vi "solar_voy_def Import (cmd_tlm).vi"(6 "Suppress Errors? (T)":bool=TRUE, 8 "error in (no error)":errorcluster, 11 "cmd_tlm.txt":path) -> (0 "error out":errorcluster, 3 "PACKETS":T1[](array[typedef]) {"last_time" format="%<%H:%M:%S%3u %m/%d/%y>T"})   [LabVIEW 2018]
doc: "This imports a command or telemetry COSMOS file into packet definitions. Refer to http://cosmosrb.com/docs/cmdtlm/\n\nDefinition tags not supported: GENERIC_WRITE/READ_CONVERSION_START/END, MACRO_APPEND_START/END"
uses:
  solar_voy_def_ctl MODIFIERS STATE.ctl
  solar_voy_def_ctl MODIFIERS UNITS.ctl
  type/solar_type Item Type.ctl
  solar_voy_def_ctl ITEM TYPE.ctl
  solar_voy_def_ctl ITEM.ctl
  solar_voy_def_ctl PACKET_ID.ctl
  solar_voy_def_ctl PACKET.ctl
  solar_voy_def_ctl MODIFIERS LIMITS.ctl
  solar_voy_def_ctl MODIFIERS CONVERSION.ctl
  solar_voy_def_ctl MODIFIERS.ctl
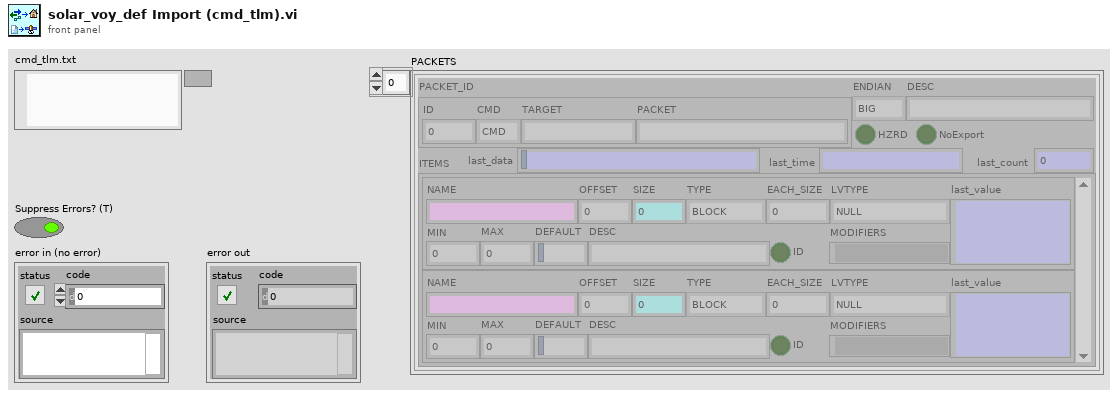
[diagram p1: front panel]
types:
  T1 = typedef "solar_voy_def_ctl PACKET.ctl" = cluster{"PACKET_ID":T2, "ENDIAN":enum8{"BIG", "LITTLE"}, "DESC":string, "HZRD":bool, "ITEMS":T3[], "NoExport":bool, "last_time":timestamp, "last_count":u32, "last_data":string}
  T2 = typedef "solar_voy_def_ctl PACKET_ID.ctl" = cluster{"ID":u16, "CMD":enum8{"CMD", "TLM"}, "TARGET":string, "PACKET":string}
  T3 = typedef "solar_voy_def_ctl ITEM.ctl" = cluster{"NAME":string, "OFFSET":i32, "SIZE":i32, "TYPE":T4, "EACH_SIZE":i32, "LVTYPE":T5, "MIN":dbl, "MAX":dbl, "DEFAULT":string, "DESC":string, "ID":bool, "MODIFIERS":variant, "last_value":variant}
  T4 = typedef "solar_voy_def_ctl ITEM TYPE.ctl" = enum8{"BLOCK", "INT", "UINT", "FLOAT", "STRING"}
  T5 = typedef "solar_type Item Type.ctl" = enum16{"NULL", "UNKNOWN", "CLUSTER", "I8", "I16", "I32", "I64", "U8", "U16", "U32", "U64", "U8_ENUM", "U16_ENUM", "U32_ENUM", "SGL", "DBL", "BOOLEAN", "STRING", "PATH", "VISA", "TAG", "TIME", "I8_1D", "I16_1D", "I32_1D", "I64_1D", "U8_1D", "U16_1D", "U32_1D", "U64_1D", "U8_ENUM_1D", "U16_ENUM_1D", "U32_ENUM_1D", "SGL_1D", "DBL_1D", "BOOLEAN_1D", "STRING_1D", "PATH_1D", "VISA_1D", "TAG_1D", "TIME_1D", "I8_2D", "I16_2D", "I32_2D", "I64_2D", "U8_2D", "U16_2D", "U32_2D", "U64_2D", "U8_ENUM_2D", "U16_ENUM_2D", "U32_ENUM_2D", "SGL_2D", "DBL_2D", "BOOLEAN_2D", "STRING_2D", "PATH_2D", "VISA_2D", "TAG_2D", "TIME_2D"}
  T6 = typedef "solar_voy_def_ctl MODIFIERS UNITS.ctl" = cluster{"FULL":string, "ABV":string}
  T7 = typedef "solar_voy_def_ctl MODIFIERS STATE.ctl" = cluster{"KEY":string, "VALUE":string, "COLOR":string, "DESC":string, "HZRD":bool}
  T8 = typedef "solar_voy_def_ctl MODIFIERS.ctl" = cluster{"LIMITS":T9, "UNITS":T6, "STATES":T7[], "CONVERSION":T10, "FORMAT":string, "REQUIRED":bool, "META":string[][]}
  T9 = typedef "solar_voy_def_ctl MODIFIERS LIMITS.ctl" = cluster{"NAME":string, "PERSIST":i32, "EN":bool, "RED_LO":dbl, "YEL_LO":dbl, "YEL_HI":dbl, "RED_HI":dbl, "GRN_LO":dbl, "GRN_HI":dbl, "FILENAME":string, "ARGS":string}
  T10 = typedef "solar_voy_def_ctl MODIFIERS CONVERSION.ctl" = cluster{"GENERIC":string, "FILENAME":string, "ARGS":string, "POLYS":cluster{"SEG":bool, "POLY":dbl[]}[]}
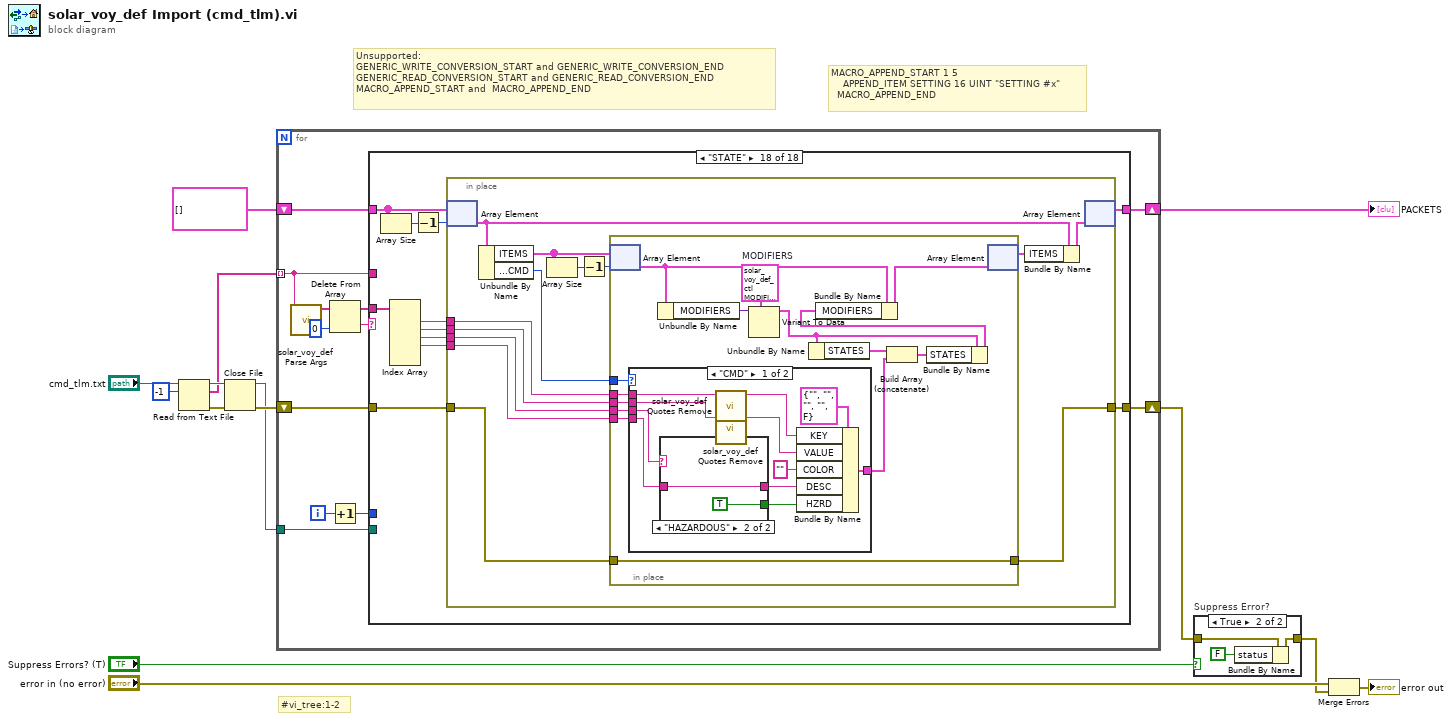
[diagram p0: block diagram]
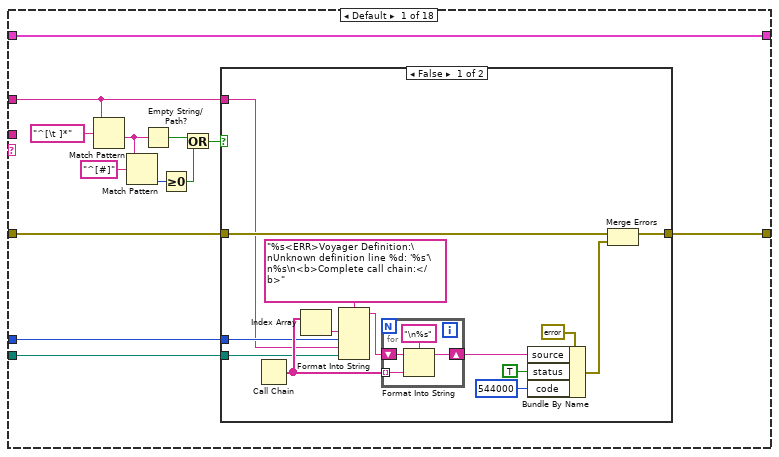
[diagram p2: hidden frame]
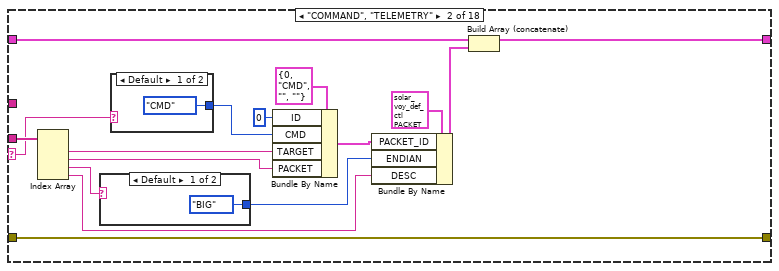
[diagram p4: hidden frame]
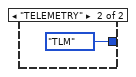
[diagram p5: hidden frame]
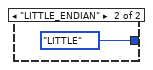
[diagram p6: hidden frame]
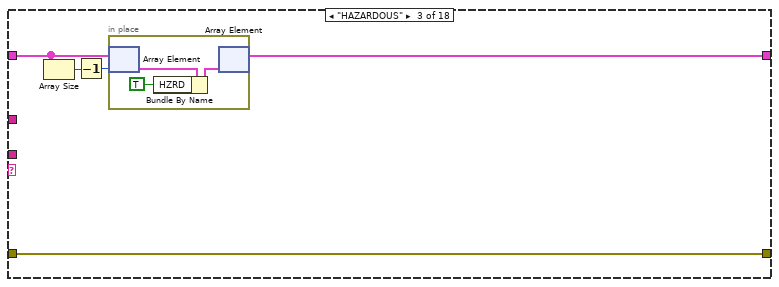
[diagram p7: hidden frame]
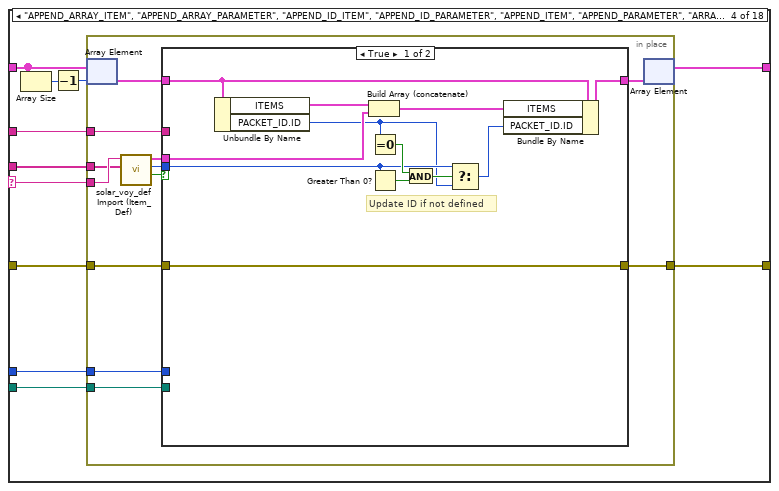
[diagram p8: hidden frame]
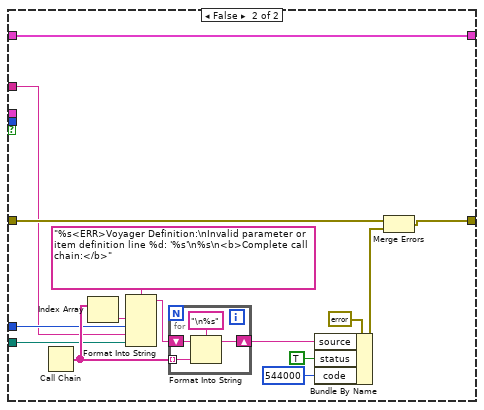
[diagram p9: hidden frame]
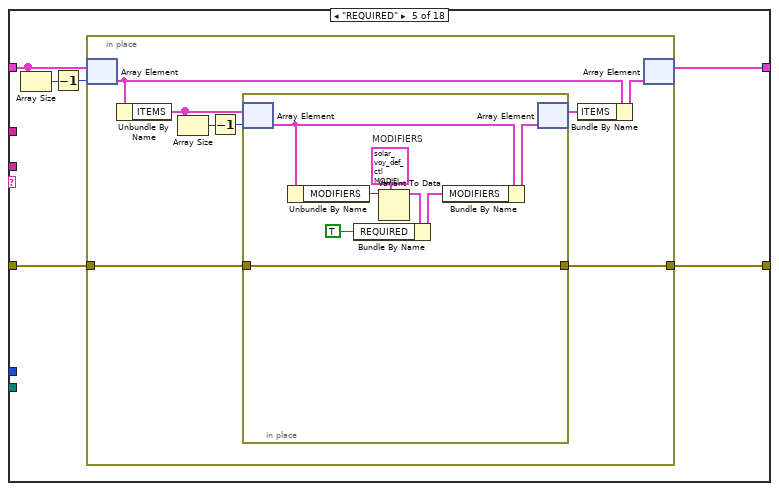
[diagram p10: hidden frame]
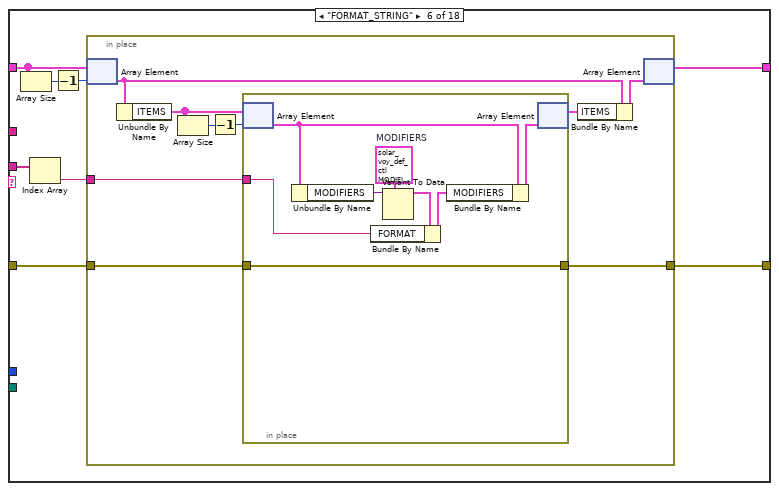
[diagram p11: hidden frame]
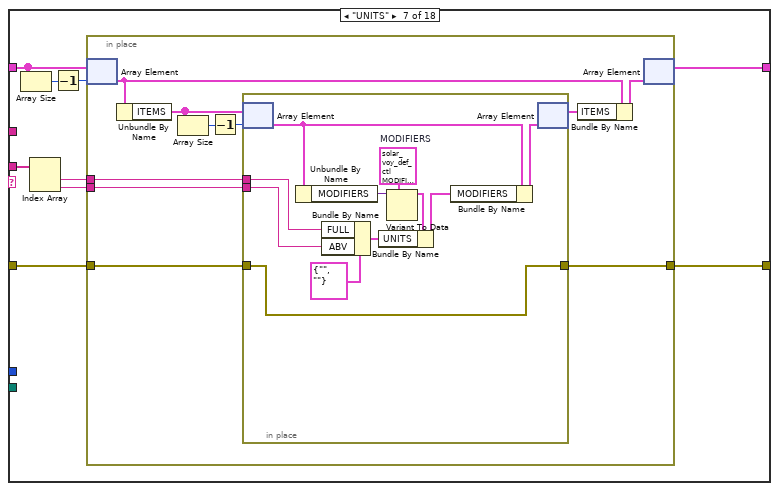
[diagram p12: hidden frame]
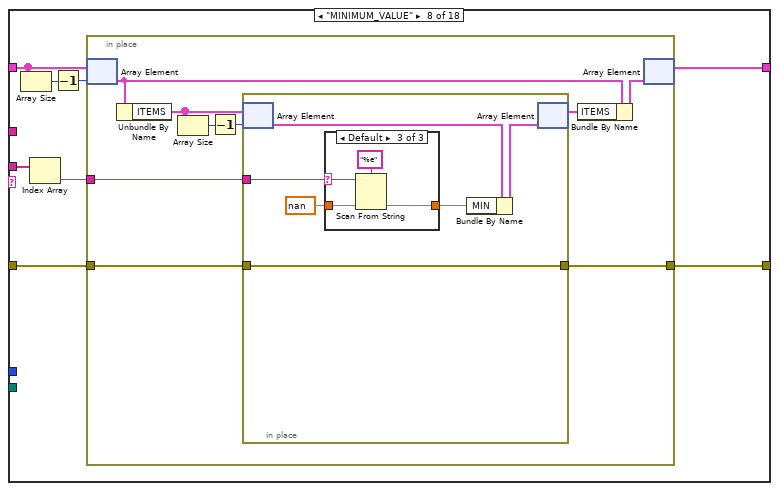
[diagram p13: hidden frame]
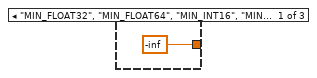
[diagram p14: hidden frame]
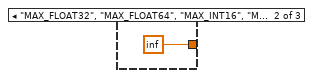
[diagram p15: hidden frame]
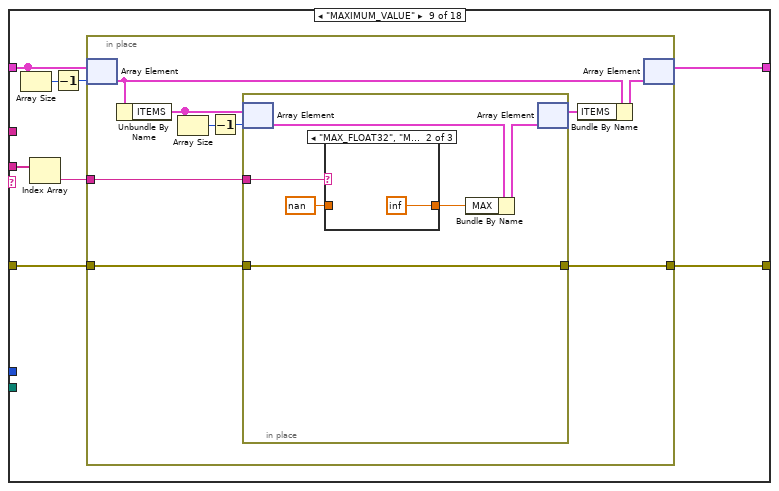
[diagram p16: hidden frame]
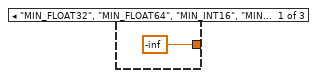
[diagram p17: hidden frame]
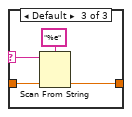
[diagram p18: hidden frame]
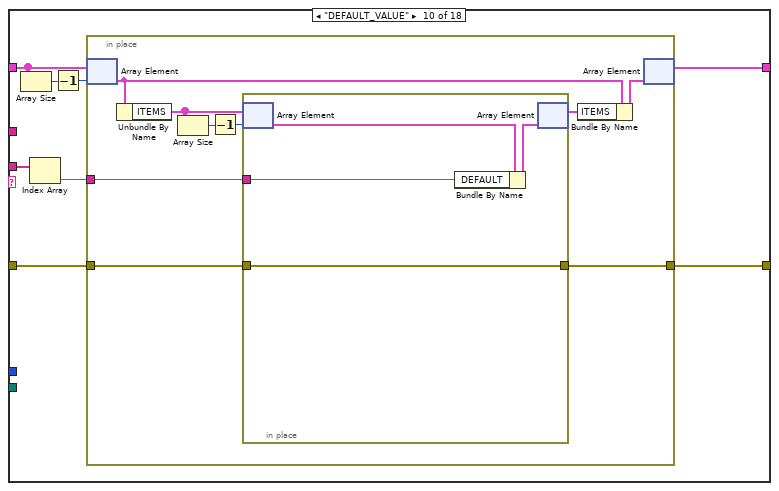
[diagram p19: hidden frame]
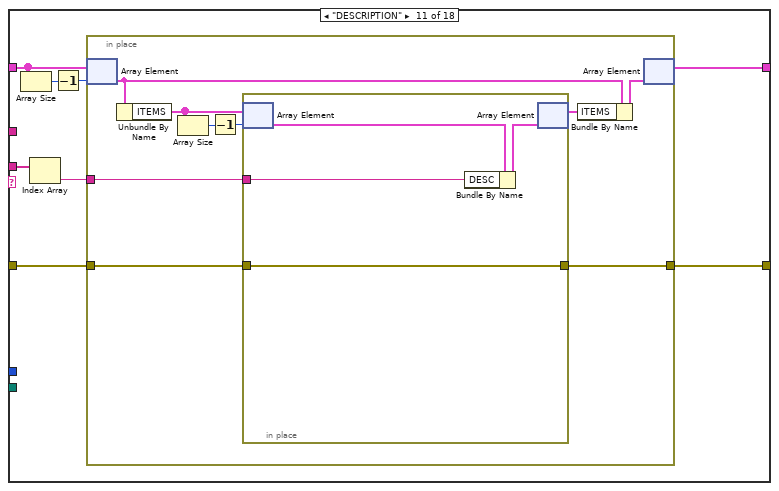
[diagram p20: hidden frame]
diagram:
  # "#vi_tree:1-2"
  # "MACRO_APPEND_START 1 5\n    APPEND_ITEM SETTING 16 UINT \"SETTING #x\"\n  MACRO_APPEND_END"
  # "Unsupported:\nGENERIC_WRITE_CONVERSION_START and GENERIC_WRITE_CONVERSION_END\nGENERIC_READ_CONVERSION_START and GENERIC_READ_CONVERSION_END\nMACRO_APPEND_START and  MACRO_APPEND_END"
  n1 = Read from Text File(file (use dialog)="cmd_tlm.txt", count=-1) -> (refnum out=w8:refnum<file>, text=w6:string[], error out=w7:errorcluster)  [unwired: 2 in, 1 out]
  n2 = Close File(refnum=w8, error in=w7) -> (path=w1:path, error out=w2:errorcluster)
  n3 = for {
    tunnel: w6 -> [w24] mode=indexing
    shift-right: [w26] -> w4
    shift-left: T1[] [] ("PACKETS") -> [w25]
    shift-right: [w23] -> w3
    shift-left: w2 -> [w22]
    tunnel: w1 -> [w17]
    i -> [w16]
    n4 = call "solar_voy_def Parse Args.vi"("String"=w24) -> ("Arguments"=w21:string[])  [unwired: 10 in]
    n5 = Delete From Array(array=w21, index=0) -> (deleted portion=w19:string, array with subset deleted=w18:string[])  [unwired: 1 in]
    n6 = Increment(x=w16) -> (x+1=w15:i32)
    n7 = case shown="\"STATE\"" w19 {
      selector: w19 -> [_ w59 _ w92 _ _ _ _ _ _ _ _ _ _ _ _ _ _]
      tunnel: [w39 w71 w80 w94 w143 w167 w193 w222 w251 w280 w301 w324 w355 w398 w452 w483 w517 w547] -> w26
      tunnel: w25 -> [w39 w72 w83 w97 w146 w170 w196 w225 w254 w283 w304 w327 w358 w401 w455 w486 w520 w550]
      tunnel: w24 -> [w34 _ _ w89 _ _ _ _ _ _ _ _ _ _ _ _ _ _]
      tunnel: [w36 w74 w79 w90 w141 w165 w191 w220 w249 w278 w299 w322 w353 w396 w450 w481 w515 w545] -> w23
      tunnel: w22 -> [w35 w74 w79 w91 w142 w166 w192 w221 w250 w279 w300 w323 w354 w397 w451 w482 w516 w546]
      tunnel: w18 -> [_ w73 _ w93 _ w164 w190 w219 w248 w277 w298 w321 w352 w395 w448 w480 w514 w544]
      tunnel: w17 -> [w38 _ _ w88 _ _ _ _ _ _ _ _ _ _ _ _ _ _]
      tunnel: w15 -> [w37 _ _ w87 _ _ _ _ _ _ _ _ _ _ _ _ _ _]
      frame Default {
        n8 = Match Pattern(string=w34, regular expression="^[\t ]*") -> (after substring=w31:string)  [unwired: 1 in, 3 out]
        n9 = Match Pattern(string=w31, regular expression="^[#]") -> (offset past match=w30:i32)  [unwired: 1 in, 3 out]
        n10 = Empty String/Path?(string/path=w31) -> (empty?=w29:bool)
        n11 = Greater Or Equal To 0?(x=w30) -> (x >= 0?=w28:bool)
        n12 = Or(x=w29, y=w28) -> (x .or. y?=w27:bool)
        n13 = case shown="False" w27 {
          tunnel: w38 -> [w44 _]
          tunnel: w37 -> [w43 _]
          tunnel: [w42 w58] -> w36
          tunnel: w35 -> [w41 w58]
          tunnel: w34 -> [w40 _]
          frame False {
            n14 = Call Chain() -> (call chain=w48:string[])
            n15 = Index Array(array=w48) -> (element=w50:string)  [unwired: 1 in]
            n16 = Format Into String(format string="%s<ERR>Voyager Definition:\nUnknown definition line %d: '%s'\n%s\n<b>Complete call chain:</b>", w50, w43, w40, w44) -> (resulting string=w49:string)  [unwired: 2 in, 1 out]
            n17 = for {
              tunnel: w48 -> [w57] mode=indexing
              shift-right: [w56] -> w47
              shift-left: w49 -> [w55]
              n18 = Format Into String(format string="\n%s", initial string=w55, w57) -> (resulting string=w56:string)  [unwired: 1 in, 1 out]
            }
            n19 = Bundle By Name(cluster=errorcluster {"status"=FALSE, "code"=0, "source"=""} ("error in (no error)"), "source"=w47, "status"=TRUE, "code"=544000 ("Code")) -> (w45:errorcluster)
            n20 = Merge Errors(w41, w45) -> (w42:errorcluster)
          }
          frame True {
            # "Empty line or comment\n- Ignore"
          }
        }
      }
      frame "COMMAND", "TELEMETRY" {
        n21 = Index Array(array=w73) -> (element #1=w70:string, element #2=w69:string, element #3=w68:string, element #4=w60:string)  [unwired: 4 in]
        n22 = case shown="Default" w68 {
          tunnel: [enum8{"BIG", "LITTLE"}."BIG" ("ENDIAN") enum8{"BIG", "LITTLE"}."LITTLE" ("ENDIAN")] -> w61
          frame Default {
          }
          frame "LITTLE_ENDIAN" {
          }
        }
        n23 = case shown="Default" w59 {
          tunnel: [enum8{"CMD", "TLM"}."CMD" ("PACKET_ID.CMD") enum8{"CMD", "TLM"}."TLM" ("PACKET_ID.CMD")] -> w67
          frame Default {
          }
          frame "TELEMETRY" {
          }
        }
        n24 = Bundle By Name(cluster=T2 {"ID"=0, "CMD"=enum."CMD", "TARGET"="", "PACKET"=""} ("PACKET_ID"), "ID"=u16 0, "CMD"=w67, "TARGET"=w70, "PACKET"=w69) -> (w62:T2)
        n25 = Bundle By Name(cluster=T1 {"PACKET_ID"={"ID"=0, "CMD"=enum."CMD", "TARGET"="", "PACKET"=""}, "ENDIAN"=enum."BIG", "DESC"="", "HZRD"=FALSE, "ITEMS"=[], "NoExport"=FALSE, "last_time"=timestamp(0 s since 1904-01-01), "last_count"=0, "last_data"=""} ("PACKET"), "PACKET_ID"=w62, "ENDIAN"=w61, "DESC"=w60) -> (w63:T1)
        n26 = Build Array (concatenate)(w72, w63) -> (w71:T1[])
      }
      frame "HAZARDOUS" {
        n27 = Array Size(array=w83) -> (size(s)=w82:i32)
        n28 = Decrement(x=w82) -> (x-1=w81:i32)
        n29 = in-place {
          n30 = in-place-array #1(w83, w81) -> (w86:T1)
          n31 = Bundle By Name(cluster=w86, "HZRD"=TRUE) -> (w85:T1)
          n32 = in-place-array #1(w85) -> (w80:T1[])  [unwired: 1 out]
        }
      }
      frame "APPEND_ARRAY_ITEM", "APPEND_ARRAY_PARAMETER", "APPEND_ID_ITEM", "APPEND_ID_PARAMETER", "APPEND_ITEM", "APPEND_PARAMETER", "ARRAY_ITEM", "ARRAY_PARAMETER", "ID_ITEM", "ID_PARAMETER", "ITEM", "PARAMETER" {
        n33 = Array Size(array=w97) -> (size(s)=w96:i32)
        n34 = Decrement(x=w96) -> (x-1=w95:i32)
        n35 = in-place {
          in-place-border: w93 -> [w105]
          in-place-border: w92 -> [w106]
          in-place-border: [w103] -> w90
          in-place-border: w91 -> [w102]
          in-place-border: w89 -> [w101]
          in-place-border: w88 -> [w100]
          in-place-border: w87 -> [w99]
          n36 = in-place-array #2(w97, w95) -> (w109:T1)
          n37 = call "solar_voy_def Import (Item_Def).vi"("Arguments"=w105, "Item Tag"=w106) -> ("Valid?"=w104:bool, "ID"=w98:u16, "ITEM"=w107:T3)  [unwired: 7 in]
          n38 = case shown="True" w104 {
            tunnel: w109 -> [w121 w125]
            tunnel: [w120 w125] -> w108
            tunnel: w107 -> [w117 _]
            tunnel: [w110 w127] -> w103
            tunnel: w102 -> [w110 w136]
            tunnel: w101 -> [_ w123]
            tunnel: w100 -> [_ w122]
            tunnel: w99 -> [_ w124]
            tunnel: w98 -> [w113 _]
            frame True {
              # "Update ID if not defined"
              n39 = Unbundle By Name(w121) -> ("ITEMS"=w119:T3[], "PACKET_ID.ID"=w112:u16)
              n40 = Build Array (concatenate)(w119, w117) -> (w118:T3[])
              n41 = Equal To 0?(x=w112) -> (x = 0?=w116:bool)
              n42 = Greater Than 0?(x=w113) -> (x > 0?=w115:bool)
              n43 = And(x=w116, y=w115) -> (x .and. y?=w114:bool)
              n44 = Select(t=w113, s=w114, f=w112) -> (s? t:f=w111:u16)
              n45 = Bundle By Name(cluster=w121, "ITEMS"=w118, "PACKET_ID.ID"=w111) -> (w120:T1)
            }
            frame False {
              n46 = Call Chain() -> (call chain=w130:string[])
              n47 = Index Array(array=w130) -> (element=w132:string)  [unwired: 1 in]
              n48 = Format Into String(format string="%s<ERR>Voyager Definition:\nInvalid parameter or item definition line %d: '%s'\n%s\n<b>Complete call chain:</b>", w132, w124, w123, w122) -> (resulting string=w131:string)  [unwired: 2 in, 1 out]
              n49 = for {
                tunnel: w130 -> [w140] mode=indexing
                shift-right: [w139] -> w129
                shift-left: w131 -> [w138]
                n50 = Format Into String(format string="\n%s", initial string=w138, w140) -> (resulting string=w139:string)  [unwired: 1 in, 1 out]
              }
              n51 = Bundle By Name(cluster=errorcluster {"status"=FALSE, "code"=0, "source"=""} ("error in (no error)"), "source"=w129, "status"=TRUE, "code"=544000 ("Code")) -> (w126:errorcluster)
              n52 = Merge Errors(w136, w126) -> (w127:errorcluster)
            }
          }
          n53 = in-place-array #2(w108) -> (w94:T1[])  [unwired: 1 out]
        }
      }
      frame "REQUIRED" {
        n54 = Array Size(array=w146) -> (size(s)=w145:i32)
        n55 = Decrement(x=w145) -> (x-1=w144:i32)
        n56 = in-place {
          in-place-border: [w148] -> w141
          in-place-border: w142 -> [w147]
          n57 = in-place-array #3(w146, w144) -> (w154:T1)
          n58 = Unbundle By Name(w154) -> ("ITEMS"=w151:T3[])
          n59 = Array Size(array=w151) -> (size(s)=w152:i32)
          n60 = Decrement(x=w152) -> (x-1=w150:i32)
          n61 = in-place {
            in-place-border: [w161] -> w148
            in-place-border: w147 -> [w161]
            w158 = T8 {"LIMITS"={"NAME"="", "PERSIST"=0, "EN"=FALSE, "RED_LO"=0.0, "YEL_LO"=0.0, "YEL_HI"=0.0, "RED_HI"=0.0, "GRN_LO"=0.0, "GRN_HI"=0.0, "FILENAME"="", "ARGS"=""}, "UNITS"={"FULL"="", "ABV"=""}, "STATES"=[], "CONVERSION"={"GENERIC"="", "FILENAME"="", "ARGS"="", "POLYS"=[]}, "FORMAT"="", "REQUIRED"=FALSE, "META"=[]}  # MODIFIERS
            n62 = in-place-array #4(w151, w150) -> (w156:T3)
            n63 = Unbundle By Name(w156) -> ("MODIFIERS"=w159:variant)
            n64 = Variant To Data(type=w158, Variant=w159) -> (data=w157:T8)  [unwired: 1 in, 1 out]
            n65 = Bundle By Name(cluster=w157, "REQUIRED"=TRUE ("MODIFIERS.REQUIRED")) -> (w155:T8)
            n66 = Bundle By Name(cluster=w156, "MODIFIERS"=w155) -> (w160:T3)
            n67 = in-place-array #4(w160) -> (w149:T3[])  [unwired: 1 out]
          }
          n68 = Bundle By Name(cluster=w154, "ITEMS"=w149) -> (w153:T1)
          n69 = in-place-array #3(w153) -> (w143:T1[])  [unwired: 1 out]
        }
      }
      frame "FORMAT_STRING" {
        n70 = Array Size(array=w170) -> (size(s)=w169:i32)
        n71 = Index Array(array=w164) -> (element=w163:string)  [unwired: 1 in]
        n72 = Decrement(x=w169) -> (x-1=w168:i32)
        n73 = in-place {
          in-place-border: [w173] -> w165
          in-place-border: w166 -> [w172]
          in-place-border: w163 -> [w171]
          n74 = in-place-array #5(w170, w168) -> (w179:T1)
          n75 = Unbundle By Name(w179) -> ("ITEMS"=w176:T3[])
          n76 = Array Size(array=w176) -> (size(s)=w177:i32)
          n77 = Decrement(x=w177) -> (x-1=w175:i32)
          n78 = in-place {
            in-place-border: [w187] -> w173
            in-place-border: w172 -> [w187]
            in-place-border: w171 -> [w186]
            w184 = T8 {"LIMITS"={"NAME"="", "PERSIST"=0, "EN"=FALSE, "RED_LO"=0.0, "YEL_LO"=0.0, "YEL_HI"=0.0, "RED_HI"=0.0, "GRN_LO"=0.0, "GRN_HI"=0.0, "FILENAME"="", "ARGS"=""}, "UNITS"={"FULL"="", "ABV"=""}, "STATES"=[], "CONVERSION"={"GENERIC"="", "FILENAME"="", "ARGS"="", "POLYS"=[]}, "FORMAT"="", "REQUIRED"=FALSE, "META"=[]}  # MODIFIERS
            n79 = in-place-array #6(w176, w175) -> (w182:T3)
            n80 = Unbundle By Name(w182) -> ("MODIFIERS"=w185:variant)
            n81 = Variant To Data(type=w184, Variant=w185) -> (data=w181:T8)  [unwired: 1 in, 1 out]
            n82 = Bundle By Name(cluster=w181, "FORMAT"=w186) -> (w180:T8)
            n83 = Bundle By Name(cluster=w182, "MODIFIERS"=w180) -> (w183:T3)
            n84 = in-place-array #6(w183) -> (w174:T3[])  [unwired: 1 out]
          }
          n85 = Bundle By Name(cluster=w179, "ITEMS"=w174) -> (w178:T1)
          n86 = in-place-array #5(w178) -> (w167:T1[])  [unwired: 1 out]
        }
      }
      frame "UNITS" {
        n87 = Array Size(array=w196) -> (size(s)=w195:i32)
        n88 = Index Array(array=w190) -> (element #1=w189:string, element #2=w188:string)  [unwired: 2 in]
        n89 = Decrement(x=w195) -> (x-1=w194:i32)
        n90 = in-place {
          in-place-border: [w200] -> w191
          in-place-border: w192 -> [w199]
          in-place-border: w189 -> [w198]
          in-place-border: w188 -> [w197]
          n91 = in-place-array #7(w196, w194) -> (w206:T1)
          n92 = Unbundle By Name(w206) -> ("ITEMS"=w203:T3[])
          n93 = Array Size(array=w203) -> (size(s)=w204:i32)
          n94 = Decrement(x=w204) -> (x-1=w202:i32)
          n95 = in-place {
            in-place-border: [w207] -> w200
            in-place-border: w199 -> [w207]
            in-place-border: w198 -> [w216]
            in-place-border: w197 -> [w215]
            w212 = T8 {"LIMITS"={"NAME"="", "PERSIST"=0, "EN"=FALSE, "RED_LO"=0.0, "YEL_LO"=0.0, "YEL_HI"=0.0, "RED_HI"=0.0, "GRN_LO"=0.0, "GRN_HI"=0.0, "FILENAME"="", "ARGS"=""}, "UNITS"={"FULL"="", "ABV"=""}, "STATES"=[], "CONVERSION"={"GENERIC"="", "FILENAME"="", "ARGS"="", "POLYS"=[]}, "FORMAT"="", "REQUIRED"=FALSE, "META"=[]}  # MODIFIERS
            n96 = in-place-array #8(w203, w202) -> (w211:T3)
            n97 = Unbundle By Name(w211) -> ("MODIFIERS"=w213:variant)
            n98 = Bundle By Name(cluster=T6 {"FULL"="", "ABV"=""} ("MODIFIERS.UNITS"), "FULL"=w216, "ABV"=w215) -> (w214:T6)
            n99 = Variant To Data(type=w212, Variant=w213) -> (data=w209:T8)  [unwired: 1 in, 1 out]
            n100 = Bundle By Name(cluster=w209, "UNITS"=w214) -> (w208:T8)
            n101 = Bundle By Name(cluster=w211, "MODIFIERS"=w208) -> (w210:T3)
            n102 = in-place-array #8(w210) -> (w201:T3[])  [unwired: 1 out]
          }
          n103 = Bundle By Name(cluster=w206, "ITEMS"=w201) -> (w205:T1)
          n104 = in-place-array #7(w205) -> (w193:T1[])  [unwired: 1 out]
        }
      }
      frame "MINIMUM_VALUE" {
        n105 = Array Size(array=w225) -> (size(s)=w224:i32)
        n106 = Index Array(array=w219) -> (element=w218:string)  [unwired: 1 in]
        n107 = Decrement(x=w224) -> (x-1=w223:i32)
        n108 = in-place {
          in-place-border: [w228] -> w220
          in-place-border: w221 -> [w227]
          in-place-border: w218 -> [w226]
          n109 = in-place-array #9(w225, w223) -> (w234:T1)
          n110 = Unbundle By Name(w234) -> ("ITEMS"=w231:T3[])
          n111 = Array Size(array=w231) -> (size(s)=w232:i32)
          n112 = Decrement(x=w232) -> (x-1=w230:i32)
          n113 = in-place {
            in-place-border: [w238] -> w228
            in-place-border: w227 -> [w238]
            in-place-border: w226 -> [w237]
            n114 = in-place-array #10(w231, w230) -> (w240:T3)
            n115 = case shown="Default" w237 {
              selector: w237 -> [_ _ w246]
              tunnel: nan ("MIN") -> [_ _ w245]
              tunnel: [-inf ("MIN") inf ("MIN") w244] -> w235
              frame "MIN_FLOAT32", "MIN_FLOAT64", "MIN_INT16", "MIN_INT32", "MIN_INT64", "MIN_INT8", "MIN_UINT16", "MIN_UINT32", "MIN_UINT64", "MIN_UINT8" {
              }
              frame "MAX_FLOAT32", "MAX_FLOAT64", "MAX_INT16", "MAX_INT32", "MAX_INT64", "MAX_INT8", "MAX_UINT16", "MAX_UINT32", "MAX_UINT64", "MAX_UINT8" {
              }
              frame Default {
                n116 = Scan From String(format string="%e", input string=w246, default 1=w245) -> (output 1=w244:dbl)  [unwired: 2 in, 3 out]
              }
            }
            n117 = Bundle By Name(cluster=w240, "MIN"=w235) -> (w239:T3)
            n118 = in-place-array #10(w239) -> (w229:T3[])  [unwired: 1 out]
          }
          n119 = Bundle By Name(cluster=w234, "ITEMS"=w229) -> (w233:T1)
          n120 = in-place-array #9(w233) -> (w222:T1[])  [unwired: 1 out]
        }
      }
      frame "MAXIMUM_VALUE" {
        n121 = Array Size(array=w254) -> (size(s)=w253:i32)
        n122 = Index Array(array=w248) -> (element=w247:string)  [unwired: 1 in]
        n123 = Decrement(x=w253) -> (x-1=w252:i32)
        n124 = in-place {
          in-place-border: [w257] -> w249
          in-place-border: w250 -> [w256]
          in-place-border: w247 -> [w255]
          n125 = in-place-array #11(w254, w252) -> (w263:T1)
          n126 = Unbundle By Name(w263) -> ("ITEMS"=w260:T3[])
          n127 = Array Size(array=w260) -> (size(s)=w261:i32)
          n128 = Decrement(x=w261) -> (x-1=w259:i32)
          n129 = in-place {
            in-place-border: [w267] -> w257
            in-place-border: w256 -> [w267]
            in-place-border: w255 -> [w266]
            n130 = in-place-array #12(w260, w259) -> (w269:T3)
            n131 = case shown="\"MAX_FLOAT32\", \"MAX_FLOAT64\", \"MAX_INT16\", \"MAX_INT32\", \"MAX_INT64\", \"MAX_INT8\", \"MAX_UINT16\", \"MAX_UINT32\", \"MAX_UINT64\", \"MAX_UINT8\"" w266 {
              selector: w266 -> [_ _ w275]
              tunnel: nan ("MIN") -> [_ _ w274]
              tunnel: [-inf ("MIN") inf ("MIN") w273] -> w264
              frame "MIN_FLOAT32", "MIN_FLOAT64", "MIN_INT16", "MIN_INT32", "MIN_INT64", "MIN_INT8", "MIN_UINT16", "MIN_UINT32", "MIN_UINT64", "MIN_UINT8" {
              }
              frame "MAX_FLOAT32", "MAX_FLOAT64", "MAX_INT16", "MAX_INT32", "MAX_INT64", "MAX_INT8", "MAX_UINT16", "MAX_UINT32", "MAX_UINT64", "MAX_UINT8" {
              }
              frame Default {
                n132 = Scan From String(format string="%e", input string=w275, default 1=w274) -> (output 1=w273:dbl)  [unwired: 2 in, 3 out]
              }
            }
            n133 = Bundle By Name(cluster=w269, "MAX"=w264) -> (w268:T3)
            n134 = in-place-array #12(w268) -> (w258:T3[])  [unwired: 1 out]
          }
          n135 = Bundle By Name(cluster=w263, "ITEMS"=w258) -> (w262:T1)
          n136 = in-place-array #11(w262) -> (w251:T1[])  [unwired: 1 out]
        }
      }
      frame "DEFAULT_VALUE" {
        n137 = Array Size(array=w283) -> (size(s)=w282:i32)
        n138 = Index Array(array=w277) -> (element=w276:string)  [unwired: 1 in]
        n139 = Decrement(x=w282) -> (x-1=w281:i32)
        n140 = in-place {
          in-place-border: [w286] -> w278
          in-place-border: w279 -> [w285]
          in-place-border: w276 -> [w284]
          n141 = in-place-array #13(w283, w281) -> (w292:T1)
          n142 = Unbundle By Name(w292) -> ("ITEMS"=w289:T3[])
          n143 = Array Size(array=w289) -> (size(s)=w290:i32)
          n144 = Decrement(x=w290) -> (x-1=w288:i32)
          n145 = in-place {
            in-place-border: [w294] -> w286
            in-place-border: w285 -> [w294]
            in-place-border: w284 -> [w293]
            n146 = in-place-array #14(w289, w288) -> (w296:T3)
            n147 = Bundle By Name(cluster=w296, "DEFAULT"=w293) -> (w295:T3)
            n148 = in-place-array #14(w295) -> (w287:T3[])  [unwired: 1 out]
          }
          n149 = Bundle By Name(cluster=w292, "ITEMS"=w287) -> (w291:T1)
          n150 = in-place-array #13(w291) -> (w280:T1[])  [unwired: 1 out]
        }
      }
      frame "DESCRIPTION" {
        n151 = Array Size(array=w304) -> (size(s)=w303:i32)
        n152 = Index Array(array=w298) -> (element=w297:string)  [unwired: 1 in]
        n153 = Decrement(x=w303) -> (x-1=w302:i32)
        n154 = in-place {
          in-place-border: [w307] -> w299
          in-place-border: w300 -> [w306]
          in-place-border: w297 -> [w305]
          n155 = in-place-array #15(w304, w302) -> (w313:T1)
          n156 = Unbundle By Name(w313) -> ("ITEMS"=w310:T3[])
          n157 = Array Size(array=w310) -> (size(s)=w311:i32)
          n158 = Decrement(x=w311) -> (x-1=w309:i32)
          n159 = in-place {
            in-place-border: [w315] -> w307
            in-place-border: w306 -> [w315]
            in-place-border: w305 -> [w314]
            n160 = in-place-array #16(w310, w309) -> (w317:T3)
            n161 = Bundle By Name(cluster=w317, "DESC"=w314) -> (w316:T3)
            n162 = in-place-array #16(w316) -> (w308:T3[])  [unwired: 1 out]
          }
          n163 = Bundle By Name(cluster=w313, "ITEMS"=w308) -> (w312:T1)
          n164 = in-place-array #15(w312) -> (w301:T1[])  [unwired: 1 out]
        }
      }
      frame "READ_CONVERSION", "WRITE_CONVERSION" {
        n165 = Array Size(array=w327) -> (size(s)=w326:i32)
        n166 = Delete From Array(array=w321, index=0) -> (deleted portion=w320:string, array with subset deleted=w318:string[])  [unwired: 1 in]
        n167 = Decrement(x=w326) -> (x-1=w325:i32)
        n168 = in-place {
          in-place-border: [w333] -> w322
          in-place-border: w323 -> [w332]
          in-place-border: w320 -> [w331]
          in-place-border: w318 -> [w330]
          n169 = in-place-array #17(w327, w325) -> (w339:T1)
          n170 = for {
            tunnel: w330 -> [w342] mode=indexing
            tunnel: [w340] -> w329 mode=indexing
            n171 = Concatenate Strings(w342, " " ("string")) -> (w340:string)
          }
          n172 = Unbundle By Name(w339) -> ("ITEMS"=w336:T3[])
          n173 = Array Size(array=w336) -> (size(s)=w337:i32)
          n174 = Decrement(x=w337) -> (x-1=w335:i32)
          n175 = Concatenate Strings(w329) -> (w328:string)
          n176 = in-place {
            in-place-border: [w351] -> w333
            in-place-border: w332 -> [w351]
            in-place-border: w331 -> [w350]
            in-place-border: w328 -> [w349]
            w347 = T8 {"LIMITS"={"NAME"="", "PERSIST"=0, "EN"=FALSE, "RED_LO"=0.0, "YEL_LO"=0.0, "YEL_HI"=0.0, "RED_HI"=0.0, "GRN_LO"=0.0, "GRN_HI"=0.0, "FILENAME"="", "ARGS"=""}, "UNITS"={"FULL"="", "ABV"=""}, "STATES"=[], "CONVERSION"={"GENERIC"="", "FILENAME"="", "ARGS"="", "POLYS"=[]}, "FORMAT"="", "REQUIRED"=FALSE, "META"=[]}  # MODIFIERS
            n177 = in-place-array #18(w336, w335) -> (w346:T3)
            n178 = Unbundle By Name(w346) -> ("MODIFIERS"=w348:variant)
            n179 = Variant To Data(type=w347, Variant=w348) -> (data=w344:T8)  [unwired: 1 in, 1 out]
            n180 = Bundle By Name(cluster=w344, "CONVERSION.FILENAME"=w350, "CONVERSION.ARGS"=w349) -> (w343:T8)
            n181 = Bundle By Name(cluster=w346, "MODIFIERS"=w343) -> (w345:T3)
            n182 = in-place-array #18(w345) -> (w334:T3[])  [unwired: 1 out]
          }
          n183 = Bundle By Name(cluster=w339, "ITEMS"=w334) -> (w338:T1)
          n184 = in-place-array #17(w338) -> (w324:T1[])  [unwired: 1 out]
        }
      }
      frame "SEG_POLY_READ_CONVERSION", "SEG_POLY_WRITE_CONVERSION" {
        n185 = Array Size(array=w358) -> (size(s)=w357:i32)
        n186 = Decrement(x=w357) -> (x-1=w356:i32)
        n187 = in-place {
          in-place-border: [w362] -> w353
          in-place-border: w354 -> [w361]
          in-place-border: w352 -> [w360]
          n188 = in-place-array #19(w358, w356) -> (w368:T1)
          n189 = for {
            tunnel: w360 -> [w372] mode=indexing
            tunnel: [w369] -> w359 mode=indexing
            n190 = Scan From String(format string="%e", input string=w372, default 1=nan ("default value 1")) -> (output 1=w369:dbl)  [unwired: 2 in, 3 out]
          }
          n191 = Unbundle By Name(w368) -> ("ITEMS"=w365:T3[])
          n192 = Array Size(array=w365) -> (size(s)=w366:i32)
          n193 = Decrement(x=w366) -> (x-1=w364:i32)
          n194 = in-place {
            in-place-border: [w379] -> w362
            in-place-border: w361 -> [w379]
            in-place-border: w359 -> [w380]
            w377 = T8 {"LIMITS"={"NAME"="", "PERSIST"=0, "EN"=FALSE, "RED_LO"=0.0, "YEL_LO"=0.0, "YEL_HI"=0.0, "RED_HI"=0.0, "GRN_LO"=0.0, "GRN_HI"=0.0, "FILENAME"="", "ARGS"=""}, "UNITS"={"FULL"="", "ABV"=""}, "STATES"=[], "CONVERSION"={"GENERIC"="", "FILENAME"="", "ARGS"="", "POLYS"=[]}, "FORMAT"="", "REQUIRED"=FALSE, "META"=[]}  # MODIFIERS
            n195 = in-place-array #20(w365, w364) -> (w376:T3)
            n196 = Unbundle By Name(w376) -> ("MODIFIERS"=w378:variant)
            n197 = Bundle By Name(cluster=cluster{"SEG":bool, "POLY":dbl[]} {"SEG"=FALSE, "POLY"=[]} ("POLY"), "SEG"=TRUE, "POLY"=w380) -> (w382:cluster{"SEG":bool, "POLY":dbl[]})
            n198 = Variant To Data(type=w377, Variant=w378) -> (data=w374:T8)  [unwired: 1 in, 1 out]
            n199 = Unbundle By Name(w374) -> ("CONVERSION.POLYS"=w385:cluster{"SEG":bool, "POLY":dbl[]}[])
            n200 = Build Array (concatenate)(w385, w382) -> (w384:cluster{"SEG":bool, "POLY":dbl[]}[])
            n201 = Bundle By Name(cluster=w374, "CONVERSION.POLYS"=w384) -> (w373:T8)
            n202 = Bundle By Name(cluster=w376, "MODIFIERS"=w373) -> (w375:T3)
            n203 = in-place-array #20(w375) -> (w363:T3[])  [unwired: 1 out]
          }
          n204 = Bundle By Name(cluster=w368, "ITEMS"=w363) -> (w367:T1)
          n205 = in-place-array #19(w367) -> (w355:T1[])  [unwired: 1 out]
        }
      }
      frame "LIMITS" {
        n206 = Array Size(array=w401) -> (size(s)=w400:i32)
        n207 = Index Array(array=w395) -> (element #1=w394:string, element #2=w393:string, element #3=w392:string, element #4=w391:string, element #5=w390:string, element #6=w389:string, element #7=w388:string, element #8=w387:string, element #9=w386:string)  [unwired: 9 in]
        n208 = Decrement(x=w400) -> (x-1=w399:i32)
        n209 = in-place {
          in-place-border: [w414] -> w396
          in-place-border: w397 -> [w413]
          in-place-border: w394 -> [w412]
          in-place-border: w393 -> [w411]
          in-place-border: w392 -> [w410]
          in-place-border: w391 -> [w409]
          in-place-border: w390 -> [w408]
          in-place-border: w389 -> [w407]
          in-place-border: w388 -> [w406]
          in-place-border: w387 -> [w405]
          in-place-border: w386 -> [w404]
          n210 = in-place-array #21(w401, w399) -> (w420:T1)
          n211 = Build Array(w409, w408, w407, w406, w405, w404) -> (w403:string[])
          n212 = Unbundle By Name(w420) -> ("ITEMS"=w417:T3[])
          n213 = for {
            tunnel: w403 -> [w424] mode=indexing
            tunnel: [w421] -> w402 mode=indexing
            n214 = Scan From String(format string="%e", input string=w424, default 1=nan ("default value 1")) -> (output 1=w421:dbl)  [unwired: 2 in, 3 out]
          }
          n215 = Array Size(array=w417) -> (size(s)=w418:i32)
          n216 = Decrement(x=w418) -> (x-1=w416:i32)
          n217 = in-place {
            in-place-border: [w444] -> w414
            in-place-border: w413 -> [w444]
            in-place-border: w412 -> [w443]
            in-place-border: w411 -> [w442]
            in-place-border: w410 -> [w439]
            in-place-border: w402 -> [w437]
            w429 = T8 {"LIMITS"={"NAME"="", "PERSIST"=0, "EN"=FALSE, "RED_LO"=0.0, "YEL_LO"=0.0, "YEL_HI"=0.0, "RED_HI"=0.0, "GRN_LO"=0.0, "GRN_HI"=0.0, "FILENAME"="", "ARGS"=""}, "UNITS"={"FULL"="", "ABV"=""}, "STATES"=[], "CONVERSION"={"GENERIC"="", "FILENAME"="", "ARGS"="", "POLYS"=[]}, "FORMAT"="", "REQUIRED"=FALSE, "META"=[]}  # MODIFIERS
            n218 = in-place-array #22(w417, w416) -> (w428:T3)
            n219 = case shown="\"ENABLED\"" w439 {
              tunnel: [_ TRUE] -> w438
              frame Default {
              }
              frame "ENABLED" {
              }
            }
            n220 = Index Array(array=w437) -> (element #1=w436:dbl, element #2=w435:dbl, element #3=w434:dbl, element #4=w433:dbl, element #5=w432:dbl, element #6=w431:dbl)  [unwired: 6 in]
            n221 = Decimal String To Number(string=w442, default (0L)=0 ("MODIFIERS.LIMITS.PERSIST")) -> (number=w440:i32)  [unwired: 1 in, 1 out]
            n222 = Unbundle By Name(w428) -> ("MODIFIERS"=w430:variant)
            n223 = Variant To Data(type=w429, Variant=w430) -> (data=w426:T8)  [unwired: 1 in, 1 out]
            n224 = Bundle By Name(cluster=w426, "LIMITS.NAME"=w443, "LIMITS.PERSIST"=w440, "LIMITS.EN"=w438, "LIMITS.RED_LO"=w436, "LIMITS.YEL_LO"=w435, "LIMITS.YEL_HI"=w434, "LIMITS.RED_HI"=w433, "LIMITS.GRN_LO"=w432, "LIMITS.GRN_HI"=w431) -> (w425:T8)
            n225 = Bundle By Name(cluster=w428, "MODIFIERS"=w425) -> (w427:T3)
            n226 = in-place-array #22(w427) -> (w415:T3[])  [unwired: 1 out]
          }
          n227 = Bundle By Name(cluster=w420, "ITEMS"=w415) -> (w419:T1)
          n228 = in-place-array #21(w419) -> (w398:T1[])  [unwired: 1 out]
        }
      }
      frame "LIMITS_RESPONSE" {
        n229 = Array Size(array=w455) -> (size(s)=w454:i32)
        n230 = Delete From Array(array=w448, index=0) -> (deleted portion=w447:string, array with subset deleted=w446:string[])  [unwired: 1 in]
        n231 = Decrement(x=w454) -> (x-1=w453:i32)
        n232 = in-place {
          in-place-border: [w461] -> w450
          in-place-border: w451 -> [w460]
          in-place-border: w447 -> [w459]
          in-place-border: w446 -> [w457]
          n233 = in-place-array #23(w455, w453) -> (w467:T1)
          n234 = for {
            tunnel: w457 -> [w470] mode=indexing
            tunnel: [w468] -> w458 mode=indexing
            n235 = Concatenate Strings(w470, " " ("string")) -> (w468:string)
          }
          n236 = Unbundle By Name(w467) -> ("ITEMS"=w464:T3[])
          n237 = Array Size(array=w464) -> (size(s)=w465:i32)
          n238 = Decrement(x=w465) -> (x-1=w463:i32)
          n239 = Concatenate Strings(w458) -> (w456:string)
          n240 = in-place {
            in-place-border: [w479] -> w461
            in-place-border: w460 -> [w479]
            in-place-border: w459 -> [w478]
            in-place-border: w456 -> [w477]
            w475 = T8 {"LIMITS"={"NAME"="", "PERSIST"=0, "EN"=FALSE, "RED_LO"=0.0, "YEL_LO"=0.0, "YEL_HI"=0.0, "RED_HI"=0.0, "GRN_LO"=0.0, "GRN_HI"=0.0, "FILENAME"="", "ARGS"=""}, "UNITS"={"FULL"="", "ABV"=""}, "STATES"=[], "CONVERSION"={"GENERIC"="", "FILENAME"="", "ARGS"="", "POLYS"=[]}, "FORMAT"="", "REQUIRED"=FALSE, "META"=[]}  # MODIFIERS
            n241 = in-place-array #24(w464, w463) -> (w472:T3)
            n242 = Unbundle By Name(w472) -> ("MODIFIERS"=w476:variant)
            n243 = Variant To Data(type=w475, Variant=w476) -> (data=w474:T8)  [unwired: 1 in, 1 out]
            n244 = Bundle By Name(cluster=w474, "LIMITS.FILENAME"=w478, "LIMITS.ARGS"=w477) -> (w473:T8)
            n245 = Bundle By Name(cluster=w472, "MODIFIERS"=w473) -> (w471:T3)
            n246 = in-place-array #24(w471) -> (w462:T3[])  [unwired: 1 out]
          }
          n247 = Bundle By Name(cluster=w467, "ITEMS"=w462) -> (w466:T1)
          n248 = in-place-array #23(w466) -> (w452:T1[])  [unwired: 1 out]
        }
      }
      frame "POLY_READ_CONVERSION", "POLY_WRITE_CONVERSION" {
        n249 = Array Size(array=w486) -> (size(s)=w485:i32)
        n250 = Decrement(x=w485) -> (x-1=w484:i32)
        n251 = in-place {
          in-place-border: [w490] -> w481
          in-place-border: w482 -> [w489]
          in-place-border: w480 -> [w488]
          n252 = in-place-array #25(w486, w484) -> (w496:T1)
          n253 = for {
            tunnel: w488 -> [w500] mode=indexing
            tunnel: [w497] -> w487 mode=indexing
            n254 = Scan From String(format string="%e", input string=w500, default 1=nan ("default value 1")) -> (output 1=w497:dbl)  [unwired: 2 in, 3 out]
          }
          n255 = Unbundle By Name(w496) -> ("ITEMS"=w493:T3[])
          n256 = Array Size(array=w493) -> (size(s)=w494:i32)
          n257 = Decrement(x=w494) -> (x-1=w492:i32)
          n258 = in-place {
            in-place-border: [w507] -> w490
            in-place-border: w489 -> [w507]
            in-place-border: w487 -> [w508]
            w505 = T8 {"LIMITS"={"NAME"="", "PERSIST"=0, "EN"=FALSE, "RED_LO"=0.0, "YEL_LO"=0.0, "YEL_HI"=0.0, "RED_HI"=0.0, "GRN_LO"=0.0, "GRN_HI"=0.0, "FILENAME"="", "ARGS"=""}, "UNITS"={"FULL"="", "ABV"=""}, "STATES"=[], "CONVERSION"={"GENERIC"="", "FILENAME"="", "ARGS"="", "POLYS"=[]}, "FORMAT"="", "REQUIRED"=FALSE, "META"=[]}  # MODIFIERS
            n259 = in-place-array #26(w493, w492) -> (w504:T3)
            n260 = Unbundle By Name(w504) -> ("MODIFIERS"=w506:variant)
            n261 = Bundle By Name(cluster=cluster{"SEG":bool, "POLY":dbl[]} {"SEG"=FALSE, "POLY"=[]} ("POLY"), "SEG"=FALSE, "POLY"=w508) -> (w510:cluster{"SEG":bool, "POLY":dbl[]})
            n262 = Variant To Data(type=w505, Variant=w506) -> (data=w502:T8)  [unwired: 1 in, 1 out]
            n263 = Unbundle By Name(w502) -> ("CONVERSION.POLYS"=w513:cluster{"SEG":bool, "POLY":dbl[]}[])
            n264 = Build Array (concatenate)(w513, w510) -> (w512:cluster{"SEG":bool, "POLY":dbl[]}[])
            n265 = Bundle By Name(cluster=w502, "CONVERSION.POLYS"=w512) -> (w501:T8)
            n266 = Bundle By Name(cluster=w504, "MODIFIERS"=w501) -> (w503:T3)
            n267 = in-place-array #26(w503) -> (w491:T3[])  [unwired: 1 out]
          }
          n268 = Bundle By Name(cluster=w496, "ITEMS"=w491) -> (w495:T1)
          n269 = in-place-array #25(w495) -> (w483:T1[])  [unwired: 1 out]
        }
      }
      frame "META" {
        n270 = Array Size(array=w520) -> (size(s)=w519:i32)
        n271 = Decrement(x=w519) -> (x-1=w518:i32)
        n272 = in-place {
          in-place-border: [w523] -> w515
          in-place-border: w516 -> [w522]
          in-place-border: w514 -> [w521]
          n273 = in-place-array #27(w520, w518) -> (w529:T1)
          n274 = Unbundle By Name(w529) -> ("ITEMS"=w526:T3[])
          n275 = Array Size(array=w526) -> (size(s)=w527:i32)
          n276 = Decrement(x=w527) -> (x-1=w525:i32)
          n277 = in-place {
            in-place-border: [w539] -> w523
            in-place-border: w522 -> [w539]
            in-place-border: w521 -> [w536]
            w534 = T8 {"LIMITS"={"NAME"="", "PERSIST"=0, "EN"=FALSE, "RED_LO"=0.0, "YEL_LO"=0.0, "YEL_HI"=0.0, "RED_HI"=0.0, "GRN_LO"=0.0, "GRN_HI"=0.0, "FILENAME"="", "ARGS"=""}, "UNITS"={"FULL"="", "ABV"=""}, "STATES"=[], "CONVERSION"={"GENERIC"="", "FILENAME"="", "ARGS"="", "POLYS"=[]}, "FORMAT"="", "REQUIRED"=FALSE, "META"=[]}  # MODIFIERS
            n278 = in-place-array #28(w526, w525) -> (w533:T3)
            n279 = Unbundle By Name(w533) -> ("MODIFIERS"=w535:variant)
            n280 = Variant To Data(type=w534, Variant=w535) -> (data=w531:T8)  [unwired: 1 in, 1 out]
            n281 = Unbundle By Name(w531) -> ("META"=w538:string[][])
            n282 = Build Array (concatenate)(w538, w536) -> (w537:string[][])
            n283 = Bundle By Name(cluster=w531, "META"=w537) -> (w530:T8)
            n284 = Bundle By Name(cluster=w533, "MODIFIERS"=w530) -> (w532:T3)
            n285 = in-place-array #28(w532) -> (w524:T3[])  [unwired: 1 out]
          }
          n286 = Bundle By Name(cluster=w529, "ITEMS"=w524) -> (w528:T1)
          n287 = in-place-array #27(w528) -> (w517:T1[])  [unwired: 1 out]
        }
      }
      frame "STATE" {
        n288 = Array Size(array=w550) -> (size(s)=w549:i32)
        n289 = Index Array(array=w544) -> (element #1=w543:string, element #2=w542:string, element #3=w541:string, element #4=w540:string)  [unwired: 6 in, 2 out]
        n290 = Decrement(x=w549) -> (x-1=w548:i32)
        n291 = in-place {
          in-place-border: [w557] -> w545
          in-place-border: w546 -> [w556]
          in-place-border: w543 -> [w555]
          in-place-border: w542 -> [w554]
          in-place-border: w541 -> [w552]
          in-place-border: w540 -> [w551]
          n292 = in-place-array #29(w550, w548) -> (w563:T1)
          n293 = Unbundle By Name(w563) -> ("ITEMS"=w560:T3[], "PACKET_ID.CMD"=w553:enum8{"CMD", "TLM"})
          n294 = Array Size(array=w560) -> (size(s)=w561:i32)
          n295 = Decrement(x=w561) -> (x-1=w559:i32)
          n296 = in-place {
            in-place-border: [w574] -> w557
            in-place-border: w556 -> [w574]
            in-place-border: w555 -> [w575]
            in-place-border: w554 -> [w573]
            in-place-border: w553 -> [w572]
            in-place-border: w552 -> [w571]
            in-place-border: w551 -> [w570]
            w568 = T8 {"LIMITS"={"NAME"="", "PERSIST"=0, "EN"=FALSE, "RED_LO"=0.0, "YEL_LO"=0.0, "YEL_HI"=0.0, "RED_HI"=0.0, "GRN_LO"=0.0, "GRN_HI"=0.0, "FILENAME"="", "ARGS"=""}, "UNITS"={"FULL"="", "ABV"=""}, "STATES"=[], "CONVERSION"={"GENERIC"="", "FILENAME"="", "ARGS"="", "POLYS"=[]}, "FORMAT"="", "REQUIRED"=FALSE, "META"=[]}  # MODIFIERS
            n297 = in-place-array #30(w560, w559) -> (w565:T3)
            n298 = case shown="\"CMD\"" w572 {
              tunnel: [w588 w602] -> w576
              tunnel: w575 -> [w582 w598]
              tunnel: w573 -> [w580 w596]
              tunnel: w571 -> [w586 w601]
              tunnel: w570 -> [w583 w600]
              frame "CMD" {
                n299 = case shown="\"HAZARDOUS\"" w586 {
                  selector: w586 -> [w590 _]
                  tunnel: [_ TRUE ("HZRD")] -> w585
                  tunnel: [w591 w593] -> w584
                  tunnel: w583 -> [w592 w593]
                  frame Default {
                    # "comment"
                    n300 = Concatenate Strings(w590, w592) -> (w591:string)
                  }
                  frame "HAZARDOUS" {
                  }
                }
                n301 = call "solar_voy_def Quotes Remove.vi"("String"=w582) -> ("String without Comments"=w581:string)  [unwired: 10 in]
                n302 = call "solar_voy_def Quotes Remove.vi"("String"=w580) -> ("String without Comments"=w579:string)  [unwired: 10 in]
                n303 = Bundle By Name(cluster=T7 {"KEY"="", "VALUE"="", "COLOR"="", "DESC"="", "HZRD"=FALSE} ("STATE"), "KEY"=w581, "VALUE"=w579, "COLOR"="", "DESC"=w584, "HZRD"=w585) -> (w588:T7)
              }
              frame "TLM" {
                n304 = call "solar_voy_def Quotes Remove.vi"("String"=w598) -> ("String without Comments"=w597:string)  [unwired: 10 in]
                n305 = call "solar_voy_def Quotes Remove.vi"("String"=w596) -> ("String without Comments"=w595:string)  [unwired: 10 in]
                n306 = Bundle By Name(cluster=T7 {"KEY"="", "VALUE"="", "COLOR"="", "DESC"="", "HZRD"=FALSE} ("STATE"), "KEY"=w597, "VALUE"=w595, "COLOR"=w601, "DESC"=w600, "HZRD"=FALSE) -> (w602:T7)
              }
            }
            n307 = Unbundle By Name(w565) -> ("MODIFIERS"=w569:variant)
            n308 = Variant To Data(type=w568, Variant=w569) -> (data=w567:T8)  [unwired: 1 in, 1 out]
            n309 = Unbundle By Name(w567) -> ("STATES"=w578:T7[])
            n310 = Build Array (concatenate)(w578, w576) -> (w577:T7[])
            n311 = Bundle By Name(cluster=w567, "STATES"=w577) -> (w566:T8)
            n312 = Bundle By Name(cluster=w565, "MODIFIERS"=w566) -> (w564:T3)
            n313 = in-place-array #30(w564) -> (w558:T3[])  [unwired: 1 out]
          }
          n314 = Bundle By Name(cluster=w563, "ITEMS"=w558) -> (w562:T1)
          n315 = in-place-array #29(w562) -> (w547:T1[])  [unwired: 1 out]
        }
      }
    }
  }
  "PACKETS" <- w4
  n316 = case "Suppress Error?" shown="True" "Suppress Errors? (T)" {
    tunnel: w3 -> [w604 w607]
    tunnel: [w604 w606] -> w12
    frame False {
    }
    frame True {
      n317 = Bundle By Name(cluster=w607, "status"=FALSE) -> (w606:errorcluster)
    }
  }
  n318 = Merge Errors("error in (no error)", w12) -> (→"error out":errorcluster)
